vi "XY Galvo Generator Underscan.vi"(0 "Exposure /ms":dbl, 1 "FOV max / V":dbl, 2 "Samples per ms":dbl, 3 "Relax /ms":dbl, 4 "FOV min/ V":dbl, 7 "Underscan /ms":dbl, 8 "Delay /ms":dbl) -> (5 "Signal":dbl[](array[numeric]))   [LabVIEW 2016]
uses:
  <vilib>/Analysis/1siggen.llb/Ramp Pattern by Samples.vi
  <vilib>/Analysis/NI_AALBase.lvlib
panel:
  out "XY Galvo":dbl[](graph)
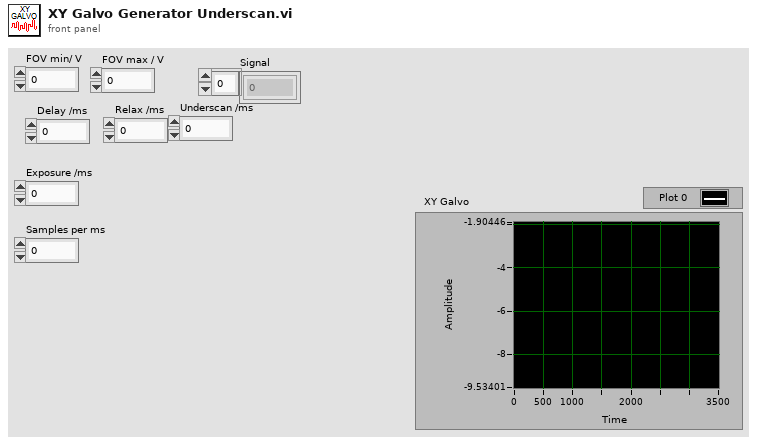
[diagram p1: front panel]
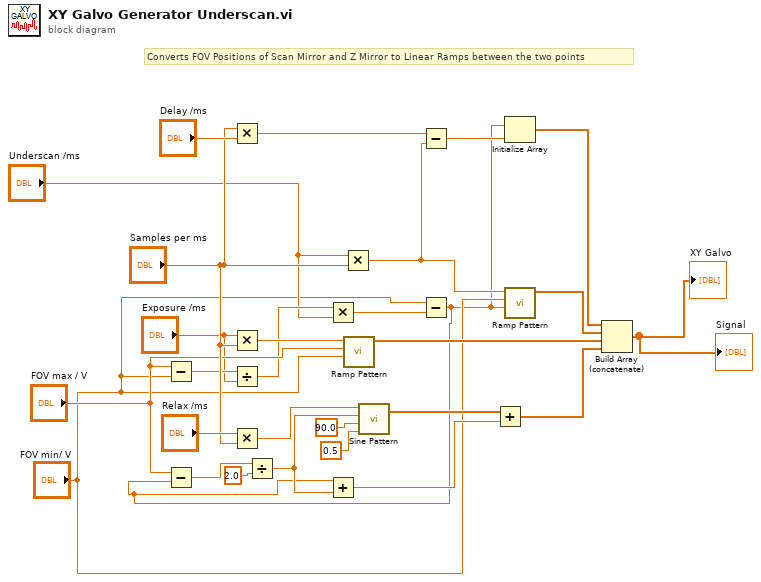
[diagram p0: block diagram]
diagram:
  # "Converts FOV Positions of Scan Mirror and Z Mirror to Linear Ramps between the two points"
  n1 = Subtract(x="FOV max / V", y="FOV min/ V") -> (x-y=w10:dbl)
  n2 = Multiply(x="Samples per ms", y="Delay /ms") -> (x*y=w8:dbl)
  n3 = Multiply(x="Exposure /ms", y="Samples per ms") -> (x*y=w21:dbl)
  n4 = Divide(x=w10, y="Exposure /ms") -> (x/y=w13:dbl)
  n5 = Multiply(x="Relax /ms", y="Samples per ms") -> (x*y=w23:dbl)
  n6 = Multiply(x=w13, y="Underscan /ms") -> (x*y=w12:dbl)
  n7 = Multiply(x="Underscan /ms", y="Samples per ms") -> (x*y=w7:dbl)
  n8 = call-poly <vilib>:"Ramp Pattern.vi"("start"="FOV min/ V", "end"="FOV max / V", "samples"=w21) -> ("Ramp Pattern"=w4:dbl[])  [unwired: 7 in, 1 out]
  n9 = Subtract(x=w8, y=w7) -> (x-y=w6:dbl)
  n10 = Subtract(x="FOV min/ V", y=w12) -> (x-y=w1:dbl)
  n11 = Subtract(x="FOV max / V", y=w1) -> (x-y=w25:dbl)
  n12 = Divide(x=w25, y=2.0 ("phase(degrees)")) -> (x/y=w28:dbl)
  n13 = Add(x=w1, y=w28) -> (x+y=w27:dbl)
  n14 = call <vilib>:"Sine Pattern.vi"("cycles"=0.5, "phase(degrees)"=90.0, "amplitude"=w28, "samples"=w23) -> ("Sinusoidal Pattern"=w19:dbl[])  [unwired: 1 out]
  n15 = Add(x=w19, y=w27) -> (x+y=w5:dbl[])
  n16 = Initialize Array(w1, w6) -> (w16:dbl[])
  n17 = call-poly <vilib>:"Ramp Pattern.vi"("start"=w1, "end"="FOV min/ V", "samples"=w7) -> ("Ramp Pattern"=w3:dbl[])  [unwired: 7 in, 1 out]
  n18 = Build Array (concatenate)(w16, w3, w4, w5) -> (→"Signal" →"XY Galvo":dbl[])
